vi "clear.vi"() -> ()   [LabVIEW 2023]
panel:
  in  "TecanPump address":u8=2
  in  "stop":bool
  in  "Valve ID":string="2"
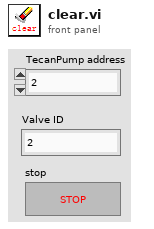
[diagram p1: front panel]
types:
  T1 = enum16{"Initialize", "Absolute Position", "Relative Pickup", "Relative Dispense", "Swich valve", "Bypass"}
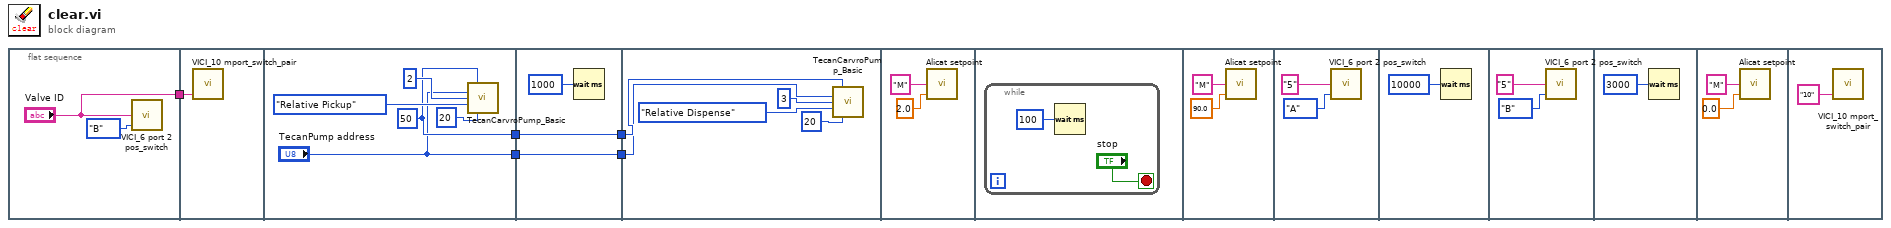
[diagram p0: block diagram]
diagram:
  n1 = flat-sequence {
    tunnel: ["Valve ID"] -> w5
    tunnel: w5 -> [w8]
    tunnel: [w10] -> w3
    tunnel: ["TecanPump address"] -> w1
    tunnel: [w15] -> w4
    tunnel: w3 -> [w15]
    tunnel: [w14] -> w2
    tunnel: w1 -> [w14]
    tunnel: w4 -> [w18]
    tunnel: w2 -> [w17]
    frame #0 {
      n2 = call "VICI_6 port 2 pos_switch.vi"("Switch to position (A/B)"=enum16{"A", "B"}."B", "Valve ID"="Valve ID") -> ()  [unwired: 2 in, 1 out]
    }
    frame #1 {
      n3 = call "VICI_10 mport_switch_pair.vi"("Go to position"=w8) -> ()  [unwired: 3 in, 1 out]
    }
    frame #2 {
      w10 = u16 50 ("Volume (μL)")
      n4 = call "TecanCarvroPump_Basic.vi"("Volume (μL)"=w10, "TecanPump address"="TecanPump address", "Valve"=u8 2, "Mode"=T1."Relative Pickup", "Speed (μL/s)"=u16 20) -> ()  [unwired: 10 in, 1 out]
    }
    frame #3 {
      n5 = Wait (ms)(milliseconds to wait=u32 1000) -> ()  [unwired: 1 out]
    }
    frame #4 {
      n6 = call "TecanCarvroPump_Basic.vi"("Volume (μL)"=w18, "TecanPump address"=w17, "Valve"=u8 3, "Mode"=T1."Relative Dispense", "Speed (μL/s)"=u16 20) -> ()  [unwired: 10 in, 1 out]
    }
    frame #5 {
      n7 = call "Alicat setpoint.vi"("Setpoint"=2.0, "Unit ID"="M") -> ()  [unwired: 3 in]
    }
    frame #6 {
      n8 = while {
        stop <- "stop" stop-if-true
        n9 = Wait (ms)(milliseconds to wait=u32 100) -> ()  [unwired: 1 out]
      }
    }
    frame #7 {
      n10 = call "Alicat setpoint.vi"("Setpoint"=90.0, "Unit ID"="M") -> ()  [unwired: 3 in]
    }
    frame #8 {
      n11 = call "VICI_6 port 2 pos_switch.vi"("Switch to position (A/B)"=enum16{"A", "B"}."A", "Valve ID"="5") -> ()  [unwired: 2 in, 1 out]
    }
    frame #9 {
      n12 = Wait (ms)(milliseconds to wait=u32 10000) -> ()  [unwired: 1 out]
    }
    frame #10 {
      n13 = call "VICI_6 port 2 pos_switch.vi"("Switch to position (A/B)"=enum16{"A", "B"}."B", "Valve ID"="5") -> ()  [unwired: 2 in, 1 out]
    }
    frame #11 {
      n14 = Wait (ms)(milliseconds to wait=u32 3000) -> ()  [unwired: 1 out]
    }
    frame #12 {
      n15 = call "Alicat setpoint.vi"("Setpoint"=0.0, "Unit ID"="M") -> ()  [unwired: 3 in]
    }
    frame #13 {
      n16 = call "VICI_10 mport_switch_pair.vi"("Go to position"="10") -> ()  [unwired: 3 in, 1 out]
    }
  }
